vi "tcp_client.vi"() -> ()   [LabVIEW 2017]
panel:
  in  "stop":bool
  in  "bytes to read":i32
  out "data out":string
  in  "Port":u16
  in  "address":string
  # "Receive Data"
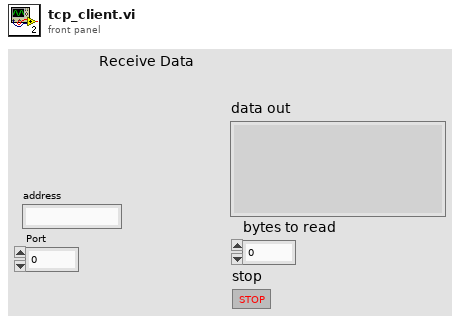
[diagram p1: front panel]
types:
  T1 = enum16{"Standard", "Buffered", "CRLF", "Immediate"}
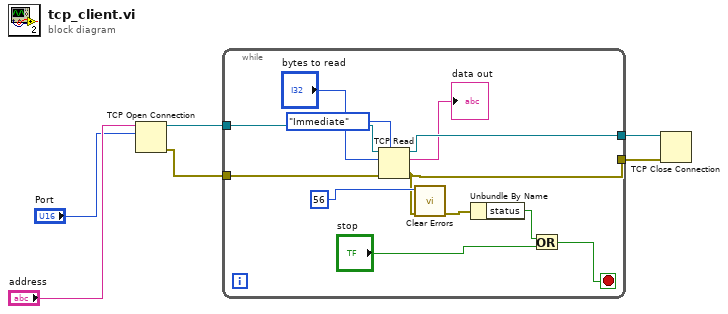
[diagram p0: block diagram]
diagram:
  n1 = TCP Open Connection(address="address", remote port or service name="Port") -> (connection ID=w2:refnum<k5>, error out=w1:errorcluster)  [unwired: 3 in]
  n2 = while {
    tunnel: [w8] -> w4
    tunnel: [w18] -> w3
    tunnel: w2 -> [w17]
    tunnel: w1 -> [w16]
    stop <- w13 stop-if-true
    n3 = TCP Read(connection ID=w17, bytes to read="bytes to read", error in (no error)=w16, 7:T1."Immediate" ("mode (standard)")) -> (connection ID out=w18:refnum<k5>, data out=→"data out":string, error out=w8:errorcluster)  [unwired: 1 in]
    n4 = call <vilib>:"Clear Errors.vi"("error in (no error)"=w8, "specific error code to clear (0: all)"=56) -> ("error out"=w7:errorcluster)  [unwired: 4 in, 1 out]
    n5 = Unbundle By Name(w7) -> ("status"=w12:bool)
    n6 = Or(x=w12, y="stop") -> (x .or. y?=w13:bool)
  }
  n7 = TCP Close Connection(connection ID=w3, error in (no error)=w4) -> ()  [unwired: 1 in, 2 out]
